vi "example.vi"() -> ()   [LabVIEW 2017]
uses:
  source/vsws_api/vsws.lvlib
panel:
  out "postdata":string
  in  "Stop Button":bool
  in  "response":string
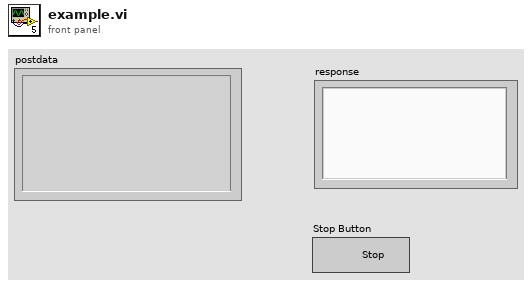
[diagram p1: front panel]
types:
  T1 = typedef "vsws.lvlib/cmdRef.ctl" = cluster{"queueRef":refnum<queue>, "reponseQueue":refnum<queue>}
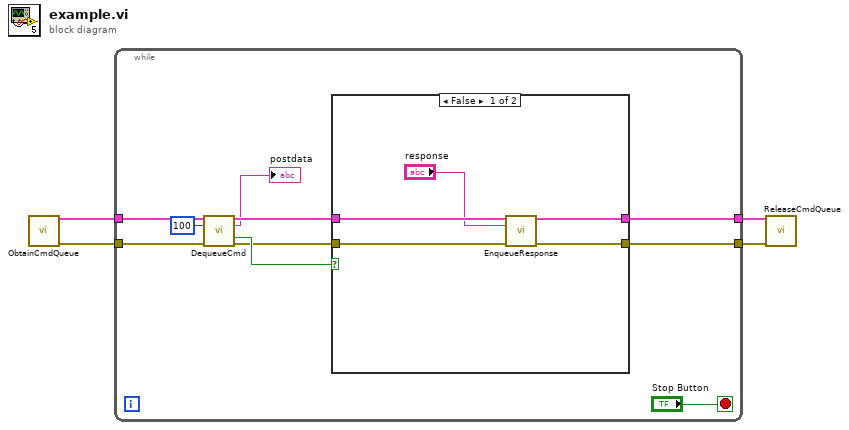
[diagram p0: block diagram]
diagram:
  n1 = call "ObtainCmdQueue.vi"() -> ("cmdRef"=w4:T1, "error out"=w3:errorcluster)  [unwired: 14 in]
  n2 = while {
    tunnel: w4 -> [w14]
    tunnel: w3 -> [w13]
    tunnel: [w8] -> w2
    tunnel: [w7] -> w1
    stop <- "Stop Button" stop-if-true
    n3 = call "DequeueCmd.vi"("cmdRef in"=w14, "timeout in ms (-1)"=100, "error in (no error)"=w13) -> ("cmdRef out"=w9:T1, "postdata"=→"postdata":string, "timed out?"=w11:bool, "error out"=w10:errorcluster)  [unwired: 9 in]
    n4 = case shown="False" w11 {
      tunnel: w10 -> [w17 w20]
      tunnel: w9 -> [w19 w21]
      tunnel: [w16 w21] -> w8
      tunnel: [w15 w20] -> w7
      frame False {
        n5 = call "EnqueueResponse.vi"("cmdRef in"=w19, "response"="response", "error in (no error)"=w17) -> ("cmdRef out"=w16:T1, "error out"=w15:errorcluster)  [unwired: 11 in]
      }
      frame True {
      }
    }
  }
  n6 = call "ReleaseCmdQueue.vi"("cmdRef"=w2, "error in (no error)"=w1) -> ()  [unwired: 13 in, 1 out]
